vi "PigeonGetStatusRates.vi"(11 "PigeonIMU DevRef In":T1={"DeviceStatus"={"status"=FALSE, "code"=0, "source"=""}, "Device Number"=0, "Type"=352321536, "Device ID"=0, "Handle"=0, "UsageFrame"=0, "Library Path"=path ""} {"Type" items=["CAN"=352321536, "TalonSRX"=33554432]}) -> (1 "PigeonIMU Get Status Rates":T3, 3 "PigeonIMU DevRef Out":T1={"DeviceStatus"={"status"=FALSE, "code"=0, "source"=""}, "Device Number"=0, "Type"=352321536, "Device ID"=0, "Handle"=0, "UsageFrame"=0, "Library Path"=path ""} {"Type" items=["CAN"=352321536, "TalonSRX"=33554432]})   [LabVIEW 2018]
uses:
  <vilib>/Rock Robotics/WPI/ThirdParty/Phoenix-LabVIEW/Pigeon IMU/CTRE_PigeonIMU_DeviceRef.ctl
  <vilib>/Rock Robotics/WPI/ThirdParty/Phoenix-LabVIEW/Pigeon IMU/CTRE_PigeonIMU_ConnectionType.ctl
  <vilib>/Rock Robotics/WPI/ThirdParty/Phoenix-LabVIEW/Pigeon IMU/CTRE_PigeonIMU_StatusFrameRate.ctl
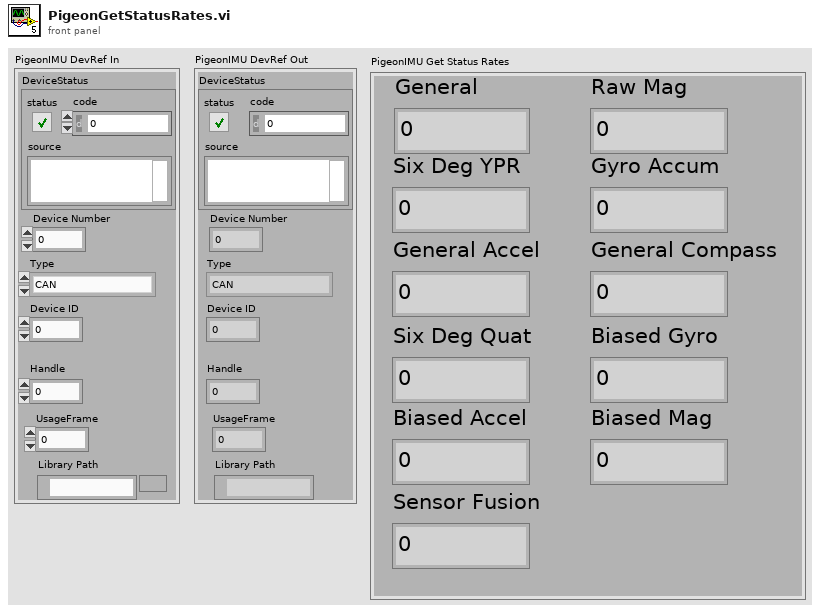
[diagram p1: front panel]
types:
  T1 = typedef "CTRE_PigeonIMU_DeviceRef.ctl" = cluster{"DeviceStatus":errorcluster, "Device Number":u8, "Type":T2, "Device ID":u32, "Handle":u64, "UsageFrame":u32, "Library Path":path}
  T2 = typedef "CTRE_PigeonIMU_ConnectionType.ctl" = u32
  T3 = cluster{"General":u32, "Six Deg YPR":u32, "Sensor Fusion":u32, "Gyro Accum":u32, "General Compass":u32, "Biased Mag":u32, "Biased Gyro":u32, "Raw Mag":u32, "Six Deg Quat":u32, "General Accel":u32, "Biased Accel":u32}
  T4 = typedef "CTRE_PigeonIMU_StatusFrameRate.ctl" = u32
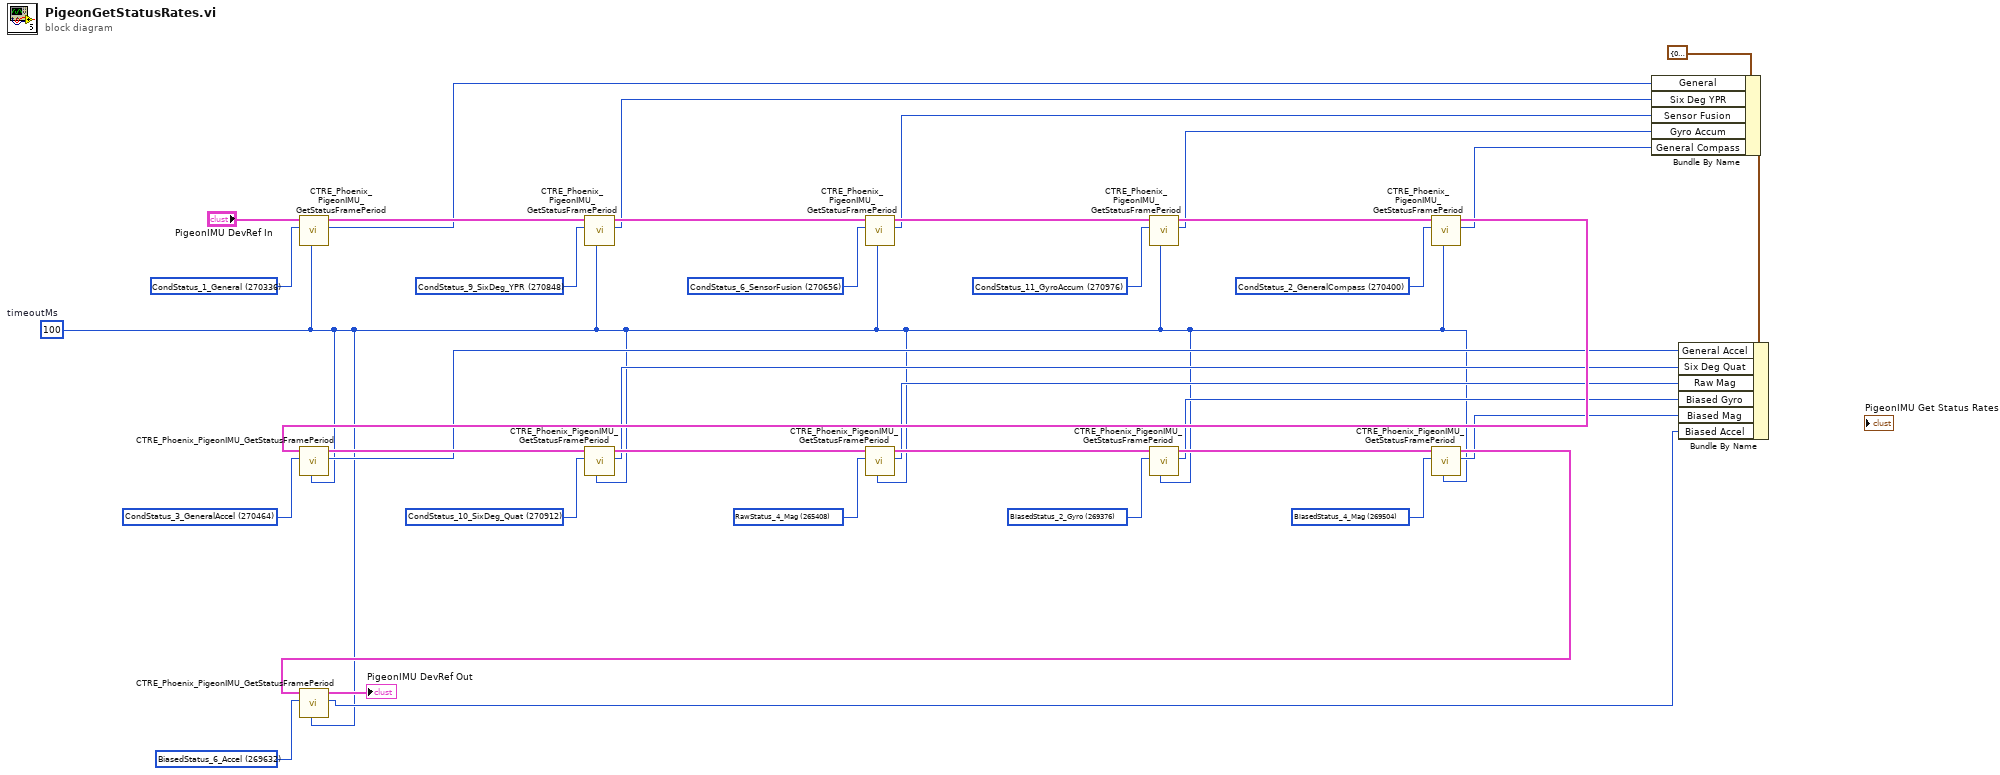
[diagram p0: block diagram]
diagram:
  w1 = u32 100  # timeoutMs
  w27 = T4 269632 items=["CondStatus_1_General"=270336, "CondStatus_9_SixDeg_YPR"=270848, "CondStatus_6_SensorFusion"=270656, "CondStatus_11_GyroAccum"=270976, "CondStatus_2_GeneralCompass"=270400, "CondStatus_3_GeneralAccel"=270464, "CondStatus_10_SixDeg_Quat"=270912, "RawStatus_4_Mag"=265408, "BiasedStatus_2_Gyro"=269376, "BiasedStatus_4_Mag"=269504, "BiasedStatus_6_Accel"=269632] ("Pigeon IMU Status Frame")
  w32 = T4 269504 items=["CondStatus_1_General"=270336, "CondStatus_9_SixDeg_YPR"=270848, "CondStatus_6_SensorFusion"=270656, "CondStatus_11_GyroAccum"=270976, "CondStatus_2_GeneralCompass"=270400, "CondStatus_3_GeneralAccel"=270464, "CondStatus_10_SixDeg_Quat"=270912, "RawStatus_4_Mag"=265408, "BiasedStatus_2_Gyro"=269376, "BiasedStatus_4_Mag"=269504, "BiasedStatus_6_Accel"=269632] ("Pigeon IMU Status Frame")
  w31 = T4 269376 items=["CondStatus_1_General"=270336, "CondStatus_9_SixDeg_YPR"=270848, "CondStatus_6_SensorFusion"=270656, "CondStatus_11_GyroAccum"=270976, "CondStatus_2_GeneralCompass"=270400, "CondStatus_3_GeneralAccel"=270464, "CondStatus_10_SixDeg_Quat"=270912, "RawStatus_4_Mag"=265408, "BiasedStatus_2_Gyro"=269376, "BiasedStatus_4_Mag"=269504, "BiasedStatus_6_Accel"=269632] ("Pigeon IMU Status Frame")
  w30 = T4 265408 items=["CondStatus_1_General"=270336, "CondStatus_9_SixDeg_YPR"=270848, "CondStatus_6_SensorFusion"=270656, "CondStatus_11_GyroAccum"=270976, "CondStatus_2_GeneralCompass"=270400, "CondStatus_3_GeneralAccel"=270464, "CondStatus_10_SixDeg_Quat"=270912, "RawStatus_4_Mag"=265408, "BiasedStatus_2_Gyro"=269376, "BiasedStatus_4_Mag"=269504, "BiasedStatus_6_Accel"=269632] ("Pigeon IMU Status Frame")
  w29 = T4 270912 items=["CondStatus_1_General"=270336, "CondStatus_9_SixDeg_YPR"=270848, "CondStatus_6_SensorFusion"=270656, "CondStatus_11_GyroAccum"=270976, "CondStatus_2_GeneralCompass"=270400, "CondStatus_3_GeneralAccel"=270464, "CondStatus_10_SixDeg_Quat"=270912, "RawStatus_4_Mag"=265408, "BiasedStatus_2_Gyro"=269376, "BiasedStatus_4_Mag"=269504, "BiasedStatus_6_Accel"=269632] ("Pigeon IMU Status Frame")
  w28 = T4 270464 items=["CondStatus_1_General"=270336, "CondStatus_9_SixDeg_YPR"=270848, "CondStatus_6_SensorFusion"=270656, "CondStatus_11_GyroAccum"=270976, "CondStatus_2_GeneralCompass"=270400, "CondStatus_3_GeneralAccel"=270464, "CondStatus_10_SixDeg_Quat"=270912, "RawStatus_4_Mag"=265408, "BiasedStatus_2_Gyro"=269376, "BiasedStatus_4_Mag"=269504, "BiasedStatus_6_Accel"=269632] ("Pigeon IMU Status Frame")
  w33 = T4 270400 items=["CondStatus_1_General"=270336, "CondStatus_9_SixDeg_YPR"=270848, "CondStatus_6_SensorFusion"=270656, "CondStatus_11_GyroAccum"=270976, "CondStatus_2_GeneralCompass"=270400, "CondStatus_3_GeneralAccel"=270464, "CondStatus_10_SixDeg_Quat"=270912, "RawStatus_4_Mag"=265408, "BiasedStatus_2_Gyro"=269376, "BiasedStatus_4_Mag"=269504, "BiasedStatus_6_Accel"=269632] ("Pigeon IMU Status Frame")
  w34 = T4 270976 items=["CondStatus_1_General"=270336, "CondStatus_9_SixDeg_YPR"=270848, "CondStatus_6_SensorFusion"=270656, "CondStatus_11_GyroAccum"=270976, "CondStatus_2_GeneralCompass"=270400, "CondStatus_3_GeneralAccel"=270464, "CondStatus_10_SixDeg_Quat"=270912, "RawStatus_4_Mag"=265408, "BiasedStatus_2_Gyro"=269376, "BiasedStatus_4_Mag"=269504, "BiasedStatus_6_Accel"=269632] ("Pigeon IMU Status Frame")
  w35 = T4 270656 items=["CondStatus_1_General"=270336, "CondStatus_9_SixDeg_YPR"=270848, "CondStatus_6_SensorFusion"=270656, "CondStatus_11_GyroAccum"=270976, "CondStatus_2_GeneralCompass"=270400, "CondStatus_3_GeneralAccel"=270464, "CondStatus_10_SixDeg_Quat"=270912, "RawStatus_4_Mag"=265408, "BiasedStatus_2_Gyro"=269376, "BiasedStatus_4_Mag"=269504, "BiasedStatus_6_Accel"=269632] ("Pigeon IMU Status Frame")
  w36 = T4 270848 items=["CondStatus_1_General"=270336, "CondStatus_9_SixDeg_YPR"=270848, "CondStatus_6_SensorFusion"=270656, "CondStatus_11_GyroAccum"=270976, "CondStatus_2_GeneralCompass"=270400, "CondStatus_3_GeneralAccel"=270464, "CondStatus_10_SixDeg_Quat"=270912, "RawStatus_4_Mag"=265408, "BiasedStatus_2_Gyro"=269376, "BiasedStatus_4_Mag"=269504, "BiasedStatus_6_Accel"=269632] ("Pigeon IMU Status Frame")
  w37 = T4 270336 items=["CondStatus_1_General"=270336, "CondStatus_9_SixDeg_YPR"=270848, "CondStatus_6_SensorFusion"=270656, "CondStatus_11_GyroAccum"=270976, "CondStatus_2_GeneralCompass"=270400, "CondStatus_3_GeneralAccel"=270464, "CondStatus_10_SixDeg_Quat"=270912, "RawStatus_4_Mag"=265408, "BiasedStatus_2_Gyro"=269376, "BiasedStatus_4_Mag"=269504, "BiasedStatus_6_Accel"=269632] ("Pigeon IMU Status Frame")
  n1 = call <vilib>:"CTRE_Phoenix_PigeonIMU_GetStatusFramePeriod.vi"("timeoutMs"=w1, "Pigeon IMU Status Frame"=w37, "CTRE_PigeonIMU_DeviceRef"="PigeonIMU DevRef In") -> ("periodMs"=w13:u32, "CTRE_PigeonIMU_DeviceRef"=w26:T1)  [unwired: 6 in, 1 out]
  n2 = call <vilib>:"CTRE_Phoenix_PigeonIMU_GetStatusFramePeriod.vi"("timeoutMs"=w1, "Pigeon IMU Status Frame"=w36, "CTRE_PigeonIMU_DeviceRef"=w26) -> ("periodMs"=w12:u32, "CTRE_PigeonIMU_DeviceRef"=w25:T1)  [unwired: 6 in, 1 out]
  n3 = call <vilib>:"CTRE_Phoenix_PigeonIMU_GetStatusFramePeriod.vi"("timeoutMs"=w1, "Pigeon IMU Status Frame"=w35, "CTRE_PigeonIMU_DeviceRef"=w25) -> ("periodMs"=w11:u32, "CTRE_PigeonIMU_DeviceRef"=w24:T1)  [unwired: 6 in, 1 out]
  n4 = call <vilib>:"CTRE_Phoenix_PigeonIMU_GetStatusFramePeriod.vi"("timeoutMs"=w1, "Pigeon IMU Status Frame"=w34, "CTRE_PigeonIMU_DeviceRef"=w24) -> ("periodMs"=w10:u32, "CTRE_PigeonIMU_DeviceRef"=w23:T1)  [unwired: 6 in, 1 out]
  n5 = call <vilib>:"CTRE_Phoenix_PigeonIMU_GetStatusFramePeriod.vi"("timeoutMs"=w1, "Pigeon IMU Status Frame"=w33, "CTRE_PigeonIMU_DeviceRef"=w23) -> ("periodMs"=w9:u32, "CTRE_PigeonIMU_DeviceRef"=w22:T1)  [unwired: 6 in, 1 out]
  n6 = call <vilib>:"CTRE_Phoenix_PigeonIMU_GetStatusFramePeriod.vi"("timeoutMs"=w1, "Pigeon IMU Status Frame"=w28, "CTRE_PigeonIMU_DeviceRef"=w22) -> ("periodMs"=w3:u32, "CTRE_PigeonIMU_DeviceRef"=w21:T1)  [unwired: 6 in, 1 out]
  n7 = call <vilib>:"CTRE_Phoenix_PigeonIMU_GetStatusFramePeriod.vi"("timeoutMs"=w1, "Pigeon IMU Status Frame"=w29, "CTRE_PigeonIMU_DeviceRef"=w21) -> ("periodMs"=w4:u32, "CTRE_PigeonIMU_DeviceRef"=w20:T1)  [unwired: 6 in, 1 out]
  n8 = call <vilib>:"CTRE_Phoenix_PigeonIMU_GetStatusFramePeriod.vi"("timeoutMs"=w1, "Pigeon IMU Status Frame"=w30, "CTRE_PigeonIMU_DeviceRef"=w20) -> ("periodMs"=w5:u32, "CTRE_PigeonIMU_DeviceRef"=w19:T1)  [unwired: 6 in, 1 out]
  n9 = call <vilib>:"CTRE_Phoenix_PigeonIMU_GetStatusFramePeriod.vi"("timeoutMs"=w1, "Pigeon IMU Status Frame"=w31, "CTRE_PigeonIMU_DeviceRef"=w19) -> ("periodMs"=w6:u32, "CTRE_PigeonIMU_DeviceRef"=w18:T1)  [unwired: 6 in, 1 out]
  n10 = call <vilib>:"CTRE_Phoenix_PigeonIMU_GetStatusFramePeriod.vi"("timeoutMs"=w1, "Pigeon IMU Status Frame"=w32, "CTRE_PigeonIMU_DeviceRef"=w18) -> ("periodMs"=w7:u32, "CTRE_PigeonIMU_DeviceRef"=w17:T1)  [unwired: 6 in, 1 out]
  n11 = call <vilib>:"CTRE_Phoenix_PigeonIMU_GetStatusFramePeriod.vi"("timeoutMs"=w1, "Pigeon IMU Status Frame"=w27, "CTRE_PigeonIMU_DeviceRef"=w17) -> ("periodMs"=w2:u32, "CTRE_PigeonIMU_DeviceRef"=→"PigeonIMU DevRef Out":T1)  [unwired: 6 in, 1 out]
  n12 = Bundle By Name(cluster=T3 {"General"=0, "Six Deg YPR"=0, "Sensor Fusion"=0, "Gyro Accum"=0, "General Compass"=0, "Biased Mag"=0, "Biased Gyro"=0, "Raw Mag"=0, "Six Deg Quat"=0, "General Accel"=0, "Biased Accel"=0} ("PigeonIMU Get Status Rates"), "General"=w13, "Six Deg YPR"=w12, "Sensor Fusion"=w11, "Gyro Accum"=w10, "General Compass"=w9) -> (w8:T3)
  n13 = Bundle By Name(cluster=w8, "General Accel"=w3, "Six Deg Quat"=w4, "Raw Mag"=w5, "Biased Gyro"=w6, "Biased Mag"=w7, "Biased Accel"=w2) -> ()  [unwired: 1 out]
